vi "Process.CheckStop.vi"(8 "error in (no error)":errorcluster, 10 "Stop Async on Error?":bool, 11 "LocalInterface.Refs":T1) -> (0 "error out":errorcluster, 3 "Stop":bool)   [LabVIEW 2025, in "bus_monitor_server_do.lvlib"]
uses:
  bus_monitor_server_do.lvlib
  Types/StreamProcess.InputRefs.ctl
  <vilib>/gRPC/LabVIEW gRPC Library/Shared/grpcId.ctl
  <vilib>/gRPC/LabVIEW gRPC Library/grpc-lvsupport-release.lvlib
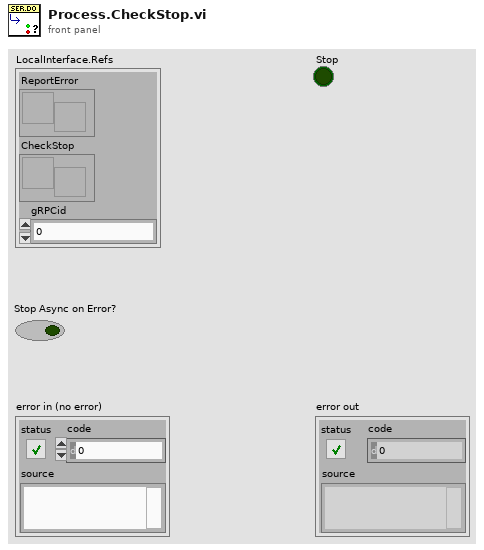
[diagram p1: front panel]
types:
  T1 = typedef "bus_monitor_server_do.lvlib/StreamProcess.InputRefs.ctl" = cluster{"ReportError":refnum<notifier>, "CheckStop":refnum<notifier>, "gRPCid":T2}
  T2 = typedef "grpc-lvsupport-release.lvlib/grpcId.ctl" = u64
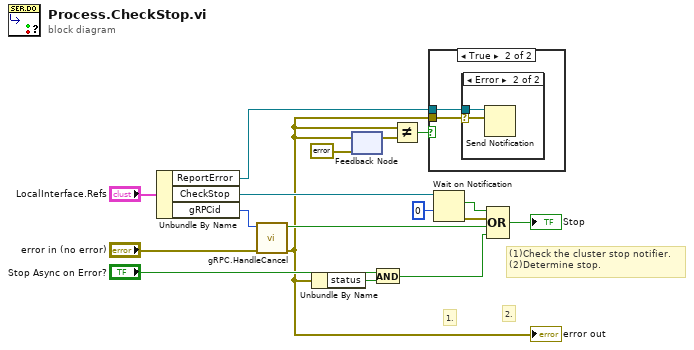
[diagram p0: block diagram]
diagram:
  # "2."
  # "1."
  # "(1)Check the cluster stop notifier.\n(2)Determine stop."
  n1 = Unbundle By Name("LocalInterface.Refs") -> ("ReportError"=w5:refnum<notifier>, "CheckStop"=w9:refnum<notifier>, "gRPCid"=w3:T2)
  n2 = call "gRPC.HandleCancel.vi"("error in (no error)"="error in (no error)", "gRPCid in"=w3) -> ("error out"=w1:errorcluster, "Stop?"=w4:bool)  [unwired: 8 in]
  "error out" <- w1
  n3 = Unbundle By Name(w1) -> ("status"=w11:bool)
  n4 = feedback #1(errorcluster {"status"=FALSE, "code"=0, "source"=""} ("Error")) -> (w7:errorcluster)
  n5 = feedback-in #1(w1) -> ()
  n6 = And(x="Stop Async on Error?", y=w11) -> (x .and. y?=w10:bool)
  n7 = Not Equal?(x=w1, y=w7) -> (x != y?=w8:bool)
  n8 = case shown="True" w8 {
    tunnel: w5 -> [_ w19]
    tunnel: w1 -> [_ w18]
    frame False {
    }
    frame True {
      n9 = case shown="Error" w18 {
        selector: w18 -> [_ w20]
        tunnel: w19 -> [_ w21]
        frame No Error {
        }
        frame Error {
          n10 = Send Notification(notification=w20, notifier=w21) -> ()  [unwired: 1 in, 2 out]
        }
      }
    }
  }
  n11 = Wait on Notification(notifier=w9, timeout in ms (-1)=0) -> (notification=w16:bool, error out=w15:errorcluster)  [unwired: 2 in, 2 out]
  n12 = Compound Arithmetic op=OR(w16, w15, w4, w10) -> (→"Stop":bool)
